vi "Don't Break the Rollers.vi"(10 "Rollers close in":bool) -> (2 "Roller close out":bool, 4 "Keeep rollers open?":bool)   [LabVIEW 2014]
uses:
  Robot Global Data.vi
panel:
  out "Keeep rollers closed?":bool
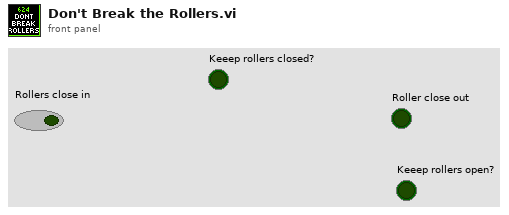
[diagram p1: front panel]
types:
  T1 = typedef "Elevator Status.ctl" = cluster{"Height":dbl, "Enc Value":dbl, "Limit Override":bool, "Mode":T2, "High IR":bool, "Motor Out":dbl, "Ping Detect":bool, "Auto Elevator Indicators":T3, "Master Current":dbl, "Slave Current":dbl, "High Current":bool, "Current Tripped":bool, "Top Limit":bool, "Bottom Limit":bool, "Eject Piston":bool, "Stabilizer":bool, "Finger":bool, "Finger Height":dbl, "Finger Raw":dbl, "Finger at Bottom":bool}
  T2 = typedef "Elevator Mode.ctl" = enum16{"Manual", "Safe", "Auto"}
  T3 = typedef "Auto Elevator Indicators.ctl" = cluster{"Target Out":dbl, "Storing Trashcan?":bool, "State":T4, "In Range":bool, "Store Can Command":bool, "HP Load":bool}
  T4 = typedef "Elevator State.ctl" = enum16{"Idle", "Goto Load Position", "Wait for Load", "Load Drop", "Load Lift", "Drop Stack", "Goto Eject Position", "Eject ", "Raise Trashcan", "Open Stabilizer", "Untip Drop", "Untip Wait", "Untip Lift", "Abort Load", "HP Load Wait", "HP Load Drop", "HP Load Lift", "HP Load Abort", "Close Stabilizer", "HP Load Unfinish", "HP Load Score", "HP Load Finish", "HP Goto Finish Down", "HP Goto Finish Up", "Full"}
  T5 = typedef "Dashboard Control Data.ctl" = cluster{"Cam Exposure":dbl, "Go to angle":dbl, "Steer PID Gains":cluster{"proportional gain (Kc)":dbl, "integral time (Ti, min)":dbl, "derivative time (Td, min)":dbl}, "Steer PID output Range":cluster{"output high":dbl, "output low":dbl}, "Pressure m \nValue":dbl, "Pressure b \nValue":dbl, "Roller Command Cluster ":T6, "Elevator":T7, "Encoder Control":T9, "Auton Settings":cluster{"Drive Dist Window Size":dbl}, "Drivetrain Settings":T10, "Lance":T11}
  T6 = typedef "Roller Control.ctl" = cluster{"Intake Speed":dbl, "Turn In Speed":dbl, "Unload Speed":dbl, "Turn Out Speed":dbl, "Ping Align Tolerance":dbl, "Tote Range Threshold":dbl, "Right Pot 0":dbl, "Pot Threshold":dbl, "Left Pot 0":dbl, "Right Pot Scale":dbl, "Left Pot Scale":dbl, "Min Elevator Height":dbl, "Eject Time":dbl, "Eject US Threshold":dbl, "Anti-Twitch Time":u32, "Ping Caring Threshold":dbl, "Pot Diff Threshold":dbl, "Pinch Sustain":u32, "Absorb Give Up Threshold":dbl, "Untip In Threshold":dbl, "Untip Grab Range":dbl, "Ultrasonic Hold Time":u32, "Landscape Absorb Time":u32, "Pot Use Wait Time":u32, "Can Turn Stop Range":dbl, "HP Load Speed":dbl, "Stick Multiplier":dbl}
  T7 = typedef "Elevator DB Control.ctl" = cluster{"PID Output Range":cluster{"output high":dbl, "output low":dbl}, "PID gains":cluster{"proportional gain (Kc)":dbl, "integral time (Ti, min)":dbl, "derivative time (Td, min)":dbl}, "Height Tolerance":sgl, " Encoder Constant":dbl, "Eject Time":sgl, "Zeroing Speed":sgl, "Presets":T8, "Ping Detect Threshold":sgl, "Trashcan Detect Threshold":sgl, "Zero Filter Time":dbl, "Stabilizer Open Time":dbl, "Zero Creep Speed":dbl, "Max Current":dbl, "Current Trip Time":dbl, "Abort Pitch":dbl, "Finger m":dbl, "Finger b":dbl, "Finger max ":dbl, "Finger Stabilizer":dbl, "Finger Store":dbl, "Finger Stop Store":dbl, "Stabilizer Close Time":dbl, "Finger min":dbl, "Unstick gain":dbl}
  T8 = typedef "Elevator Presets.ctl" = cluster{"Pickup 2 w/ Tote":sgl, "Pickup 2 w/ Trashcan":sgl, "Pickup 3 w/ Tote":sgl, "Pickup 3 w/ Trashcan":sgl, "Bottom":sgl, "Pickup 1 w/ Tote":sgl, "Pickup Trashcan":sgl, "Pickup 1 w/ Trashcan":sgl, "Eject":sgl, "Hold Low":sgl, "Step add height":sgl, "Untip Lift":dbl, "Drop Stack":dbl, "HP Load Hold":dbl, "HP Load Drop":dbl, "HP Load Hold Can":dbl, "Store can max":dbl, "HP Drag Score":dbl, "HP Drag Finish":dbl, "Finger trashcan avoid":dbl, "Full":dbl}
  T9 = typedef "Encoder Control.ctl" = cluster{"Left Tick Constant":dbl, "Right Tick Constant":dbl, "Center Tick Constant":dbl, "Reset?":bool, "Y Dist":cluster{"PID gains":cluster{"proportional gain (Kc)":dbl, "integral time (Ti, min)":dbl, "derivative time (Td, min)":dbl}}, "X Dist":cluster{"PID gains":cluster{"proportional gain (Kc)":dbl, "integral time (Ti, min)":dbl, "derivative time (Td, min)":dbl}}, "Y Stop Thresh":dbl, "Y Stop Speed":dbl, "X Stop Thresh":dbl, "X Stop Speed":dbl}
  T10 = typedef "Drivetrain Settings.ctl" = cluster{"Gyro Tolerance":sgl, "Strafe Correct max steer":sgl, "Strafe Timer Wait":sgl, "Throttle Ramp (ms)":sgl, "Strafe Ramp (ms)":sgl, "Angular rate compensation":bool, "Throttle to Rate Scale":sgl, "Rate compensation gain":sgl, "Creep Steer":sgl, "Creep Throttle":sgl}
  T11 = typedef "Pike DB Controls.ctl" = cluster{"Down Speed":dbl, "Up Speed":dbl, "Max Down Time":dbl, "Max Up Time":dbl, "Current Limit":dbl}
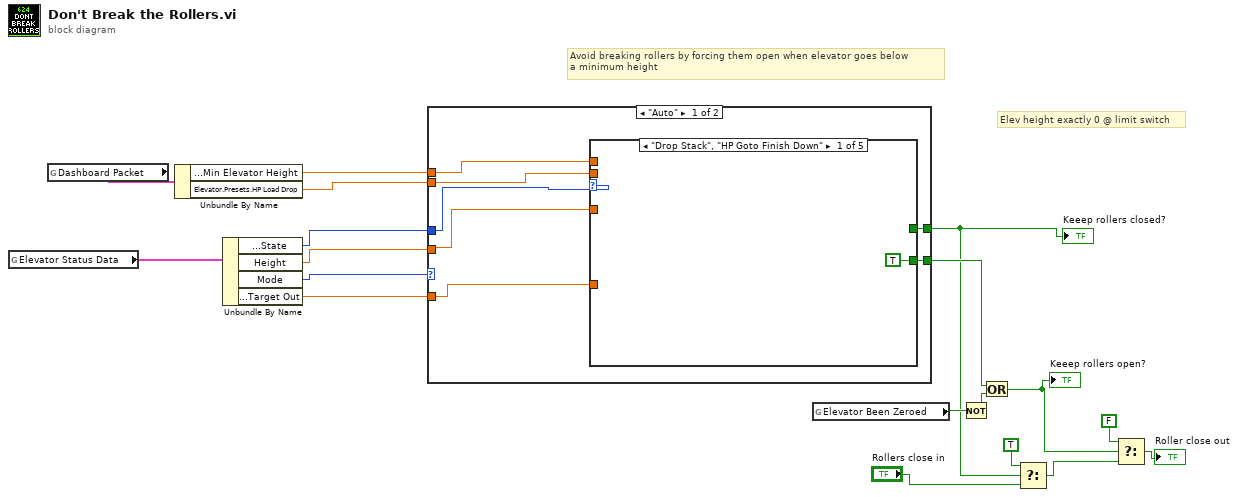
[diagram p0: block diagram]
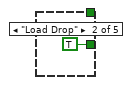
[diagram p2: hidden frame]
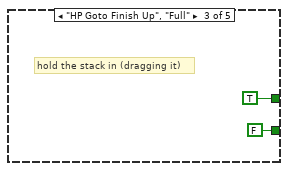
[diagram p3: hidden frame]
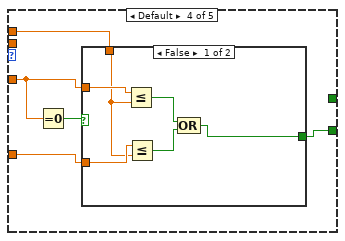
[diagram p4: hidden frame]
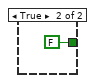
[diagram p5: hidden frame]
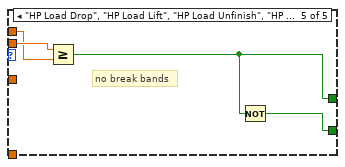
[diagram p6: hidden frame]
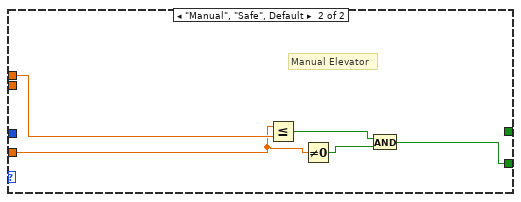
[diagram p7: hidden frame]
diagram:
  # "Elev height exactly 0 @ limit switch"
  # "Avoid breaking rollers by forcing them open when elevator goes below\na minimum height"
  n1 = global read "Robot Global Data.vi" "Elevator Status Data"() -> (w16:T1)
  n2 = global read "Robot Global Data.vi" "Dashboard Packet"() -> (w14:T5)
  n3 = Unbundle By Name(w14) -> ("Roller Command Cluster.Min Elevator Height"=w13:dbl, "Elevator.Presets.HP Load Drop"=w1:dbl)
  n4 = Unbundle By Name(w16) -> ("Auto Elevator Indicators.State"=w8:T4, "Height"=w12:dbl, "Mode"=w15:T2, "Auto Elevator Indicators.Target Out"=w7:dbl)
  n5 = case shown="\"Auto\"" w15 {
    tunnel: w13 -> [w24 w50]
    tunnel: w12 -> [w23 w48]
    tunnel: [w25 w46] -> w9
    tunnel: w8 -> [w21 _]
    tunnel: w7 -> [w22 _]
    tunnel: [w20 _] -> w3
    tunnel: w1 -> [w19 _]
    frame "Auto" {
      n6 = case shown="\"Drop Stack\", \"HP Goto Finish Down\"" w21 {
        tunnel: [TRUE TRUE FALSE w34 w44] -> w25
        tunnel: w24 -> [_ _ _ w33 w42]
        tunnel: w23 -> [_ _ _ w32 _]
        tunnel: w22 -> [_ _ _ w30 _]
        tunnel: [_ _ TRUE _ w43] -> w20
        tunnel: w19 -> [_ _ _ _ w45]
        frame "Drop Stack", "HP Goto Finish Down" {
        }
        frame "Load Drop" {
        }
        frame "HP Goto Finish Up", "Full" {
          # "hold the stack in (dragging it)"
        }
        frame Default {
          n7 = Equal To 0?(x=w32) -> (x = 0?=w31:bool)
          n8 = case shown="False" w31 {
            tunnel: w32 -> [w40 _]
            tunnel: w30 -> [w39 _]
            tunnel: w33 -> [w38 _]
            tunnel: [w35 FALSE] -> w34
            frame False {
              n9 = Less Or Equal?(x=w40, y=w38) -> (x <= y?=w37:bool)
              n10 = Less Or Equal?(x=w39, y=w38) -> (x <= y?=w36:bool)
              n11 = Compound Arithmetic op=OR(w37, w36) -> (w35:bool)
            }
            frame True {
            }
          }
        }
        frame "HP Load Drop", "HP Load Lift", "HP Load Unfinish", "HP Load Score" {
          # "no break bands"
          n12 = Greater Or Equal?(x=w45, y=w42) -> (x >= y?=w43:bool)
          n13 = Not(x=w43) -> (.not. x?=w44:bool)
        }
      }
    }
    frame "Manual", "Safe", Default {
      # "Manual Elevator"
      n14 = Less Or Equal?(x=w48, y=w50) -> (x <= y?=w49:bool)
      n15 = Not Equal To 0?(x=w48) -> (x != 0?=w47:bool)
      n16 = And(x=w49, y=w47) -> (x .and. y?=w46:bool)
    }
  }
  "Keeep rollers closed?" <- w3
  n17 = global read "Robot Global Data.vi" "Elevator Been Zeroed"() -> (w11:bool)
  n18 = Not(x=w11) -> (.not. x?=w10:bool)
  n19 = Or(x=w9, y=w10) -> (x .or. y?=w6:bool)
  "Keeep rollers open?" <- w6
  n20 = Select(t=TRUE, s=w3, f="Rollers close in") -> (s? t:f=w2:bool)
  n21 = Select(t=FALSE, s=w6, f=w2) -> (s? t:f=→"Roller close out":bool)
